vi "仪器运行状态写入.vi"(8 "error in (no error)":errorcluster caption="错误输入（无错误）", 10 "仪器状态":bool, 11 "TimingControl 输入":refnum<class "TimingControl.lvclass">) -> (0 "error out":errorcluster caption="错误输出", 3 "TimingControl 输出":refnum<class "TimingControl.lvclass">)   [LabVIEW 2016, in "ZKTimingControl.lvlib" / "TimingControl.lvclass"]
uses:
  TimingControl.lvclass
  TimingControl.lvclass/TimingControl.ctl
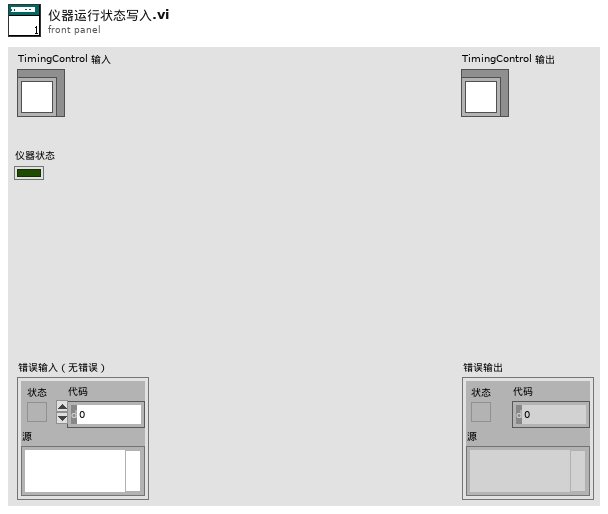
[diagram p1: front panel]
types:
  T1 = typedef "ZKTimingControl.lvlib/TimingControl.lvclass/State Data.ctl" = cluster{"仪器时间":timestamp, "仪器运行状态":bool, "配置文件路径":path, "测量参数":T2, "测试状态":cluster{"启动时间":timestamp, "结束时间":timestamp, "启动次数":dbl}, "配置信息":T3}
  T2 = typedef "ZKTimingControl.lvlib/TimingControl.lvclass/测量参数.ctl" = cluster{"氨氮":bool, "总磷":bool, "总氮":bool, "CODMn":bool, "CODCr":bool, "氟化物":bool, "挥发酚":bool}
  T3 = typedef "ZKTimingControl.lvlib/TimingControl.lvclass/配置信息.ctl" = cluster{"每周启动":T4, "每月启动":T5, "周期模式":T6, "测量参数":T2, "定点周期":T7, "间隔启动":T9, "配置时间":timestamp}
  T4 = typedef "ZKTimingControl.lvlib/TimingControl.lvclass/每周启动.ctl" = enum16{"关闭", "周日", "周一", "周二", "周三", "周四", "周五", "周六"}
  T5 = typedef "ZKTimingControl.lvlib/TimingControl.lvclass/每月启动.ctl" = enum16{"关闭", "1号", "2号", "3号", "4号", "5号", "6号", "7号", "8号", "9号", "10号", "11号", "12号", "13号", "14号", "15号", "16号", "17号", "18号", "19号", "20号", "21号", "22号", "23号", "24号", "25号", "26号", "27号", "28号", "29号", "30号", "31号"}
  T6 = typedef "ZKTimingControl.lvlib/TimingControl.lvclass/周期模式设置.ctl" = enum16{"不启用", "定点模式", "间隔模式"}
  T7 = typedef "ZKTimingControl.lvlib/TimingControl.lvclass/定点周期设置.ctl" = cluster{"启动命令":T8, "启动命令 2":T8, "启动命令 3":T8, "启动命令 4":T8, "启动命令 5":T8, "启动命令 6":T8, "启动命令 7":T8, "启动命令 8":T8, "启动命令 9":T8, "启动命令 10":T8, "启动命令 11":T8, "启动命令 12":T8, "启动命令 13":T8, "启动命令 14":T8, "启动命令 15":T8, "启动命令 16":T8, "启动命令 17":T8, "启动命令 18":T8, "启动命令 19":T8, "启动命令 20":T8, "启动命令 21":T8, "启动命令 22":T8, "启动命令 23":T8, "启动命令 24":T8}
  T8 = typedef "ZKTimingControl.lvlib/TimingControl.lvclass/启动命令选择.ctl" = enum16{"", "加标回收（启动采配水）", "加标回收（不启动采配水）", "水样测试（启动采配水）", "水样测试（不启动采配水）", "平行样测试（启动采配水）", "平行样测试（不启动采配水）", "集成干预测试"}
  T9 = typedef "ZKTimingControl.lvlib/TimingControl.lvclass/间隔启动设置.ctl" = cluster{"启动命令":T8, "启动间隔":dbl, "启动次数":i32}
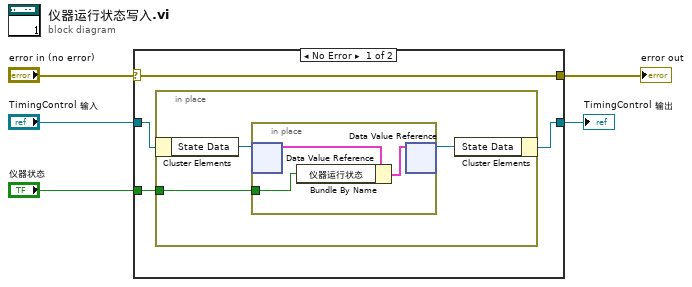
[diagram p0: block diagram]
diagram:
  n1 = case shown="No Error" "error in (no error)" {
    selector: "error in (no error)" -> [w9 w17]
    tunnel: [w9 w17] -> w4
    tunnel: [w6 w16] -> w2
    tunnel: "TimingControl 输入" -> [w8 w16]
    tunnel: "仪器状态" -> [w7 _]
    frame No Error {
      n2 = in-place {
        in-place-border: w7 -> [w11]
        n3 = in-place-cluster #1(w8) -> ("State Data"=w12:refnum<data-value>)
        n4 = in-place {
          in-place-border: w11 -> [w13]
          n5 = in-place-dvr #2(w12) -> (w15:T1)  [unwired: 1 out]
          n6 = Bundle By Name(cluster=w15, "仪器运行状态"=w13) -> (w14:T1)
          n7 = in-place-dvr #2(w14) -> (w10:refnum<data-value>)  [unwired: 1 out]
        }
        n8 = in-place-cluster #1("State Data"=w10) -> (w6:refnum<class "TimingControl.lvclass">)
      }
    }
    frame Error {
    }
  }
  "error out" <- w4
  "TimingControl 输出" <- w2
